vi "Generate Update Waveform.vi"(0 "updated signal in":refnum<class "SV Signal.lvclass">, 5 "previous signal":refnum<class "SV Signal.lvclass">, 7 "template waveform":waveform(dbl), 9 "samples":i32=1000, 11 "error in (no error)":errorcluster) -> (4 "updated signal out":refnum<class "SV Signal.lvclass">, 6 "previous signal out":refnum<class "SV Signal.lvclass">, 8 "output waveform":waveform(dbl), 10 "samples generated":i32=1000, 15 "error out":errorcluster)   [LabVIEW 2017, in "SV Signal.lvclass"]
uses:
  <vilib>/addons/_NISVFA/_Generation/Signal Generation/SV Signal/SV Signal.lvclass
  <vilib>/addons/_NISVFA/_Generation/Signal Generation/SV Signal/SV Signal.lvclass/SV Signal.ctl
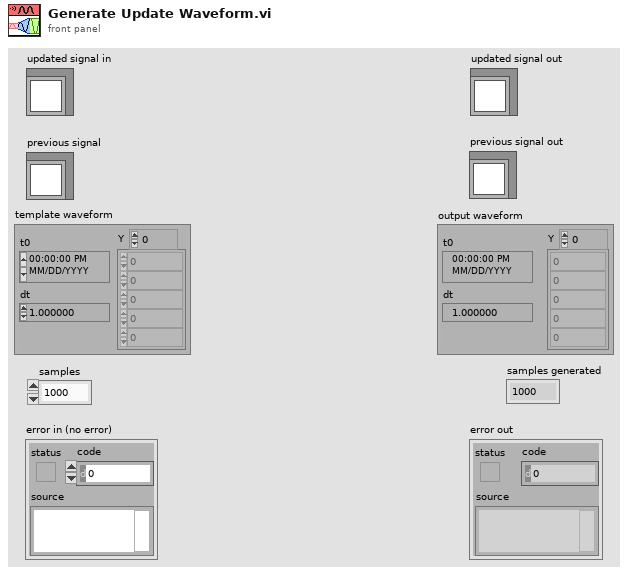
[diagram p1: front panel]
types:
  T1 = typedef "SV Signal.lvclass/sv_Generation State.ctl" = enum16{"Idle", "Ramp Up", "Pre-Measurement Settling", "Measurement", "Post-Measurement Settling", "Discrete Sweep Transition", "Ramp Down", "Update"}
  T2 = typedef "SV Signal.lvclass/sv_System Timing Model.ctl" = i64
  T3 = cluster{"system timing model":T2, "state":cluster{"RESET":bool, "generator timestamp":timestamp, "elapsed seconds":dbl, "elapsed samples":u64, "generation state":T1, "time offset at state":dbl, "samples generated at state":u64, "signal state":variant}, "duration of state":dbl, "samples remaining at state":i32}
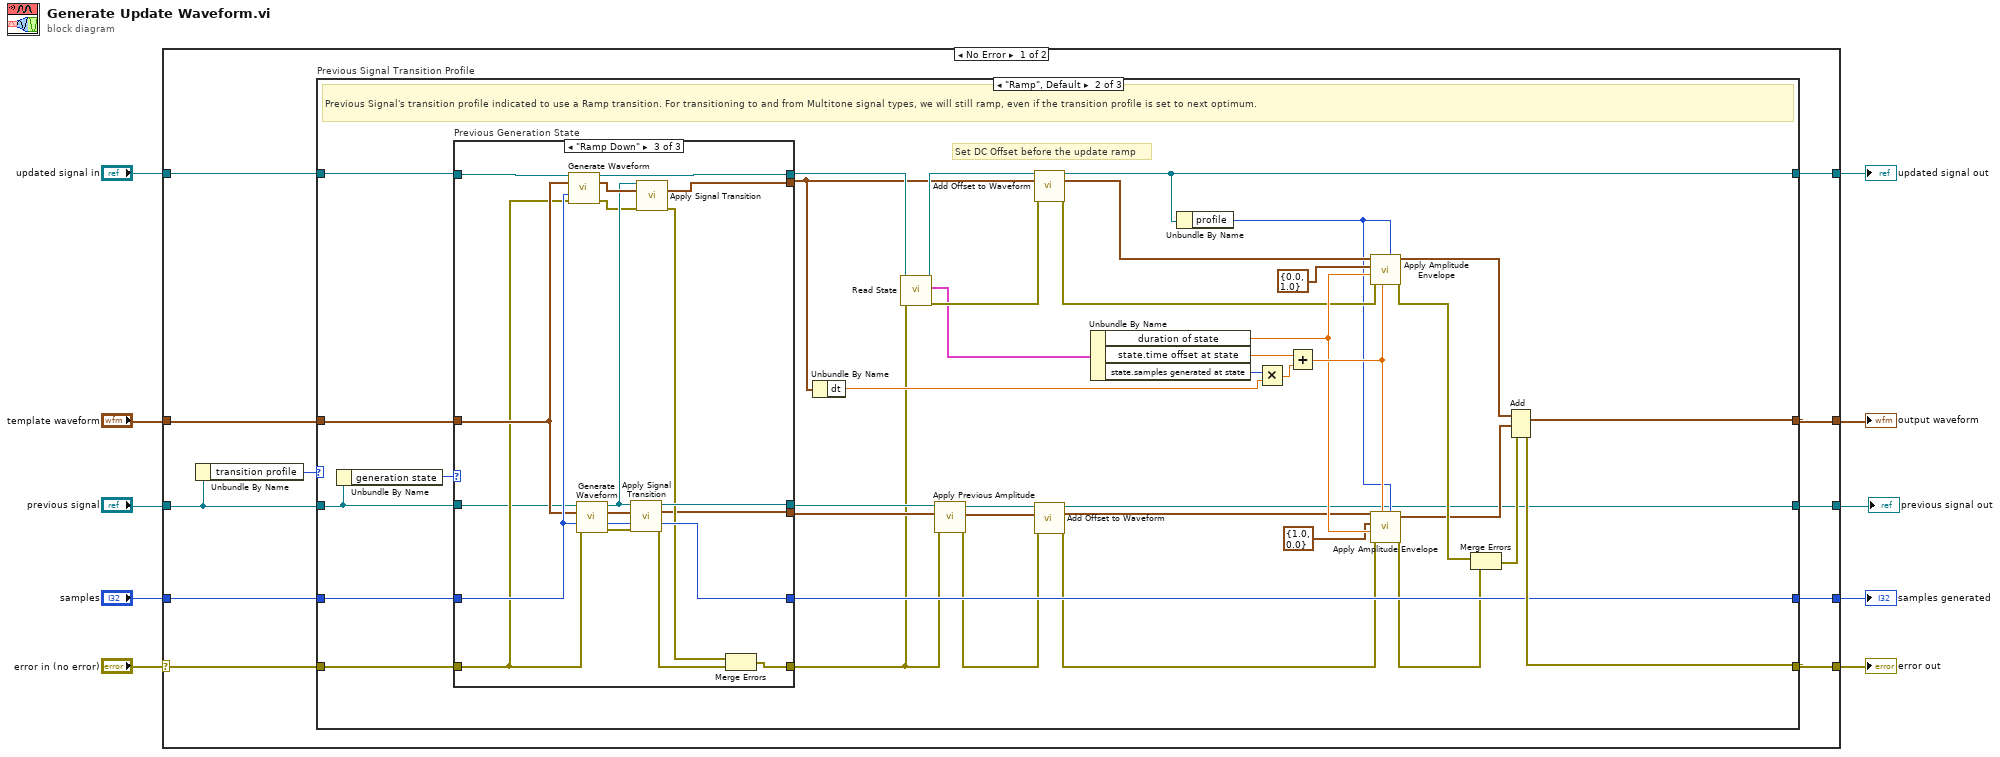
[diagram p0: block diagram]
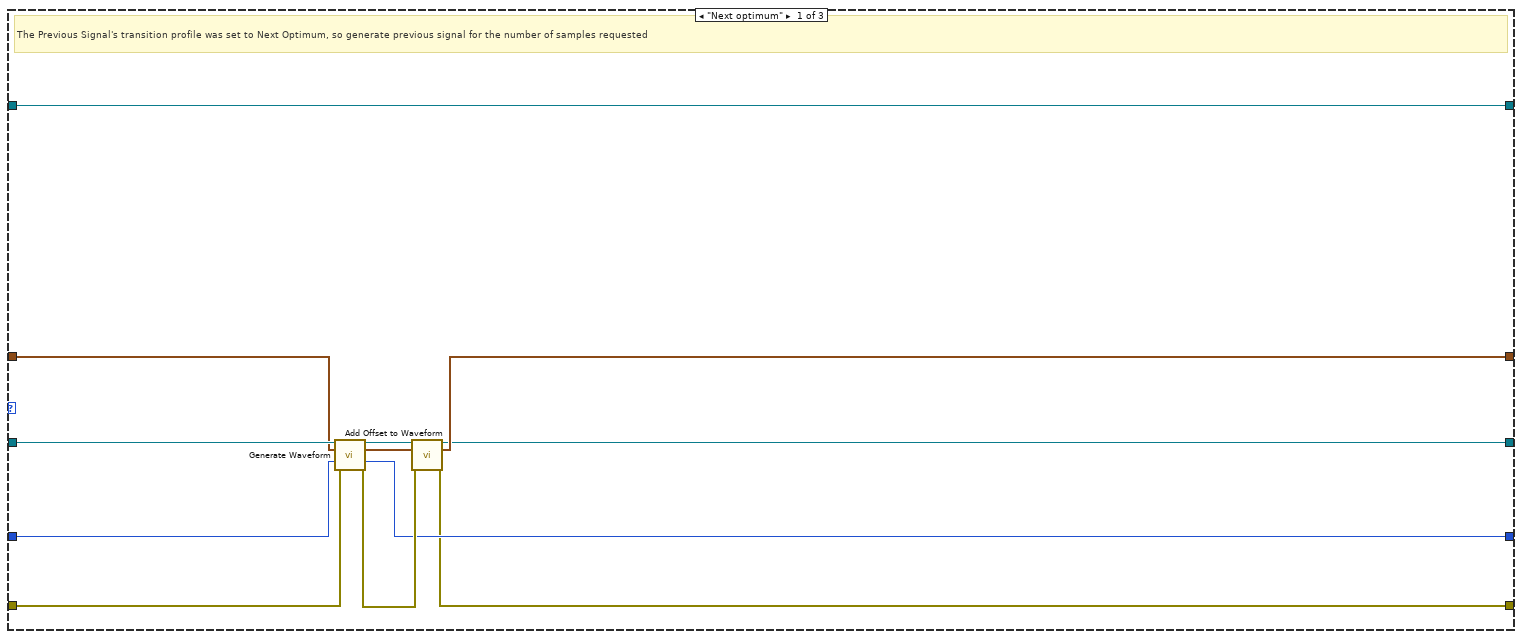
[diagram p2: hidden frame]
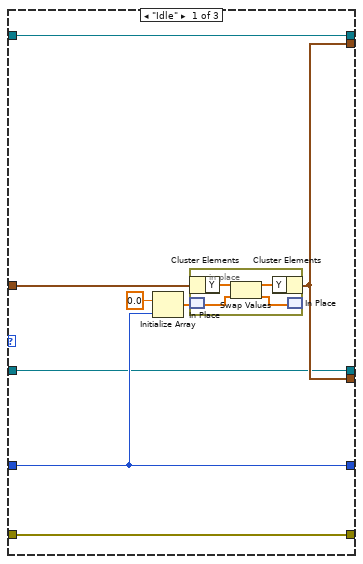
[diagram p3: hidden frame]
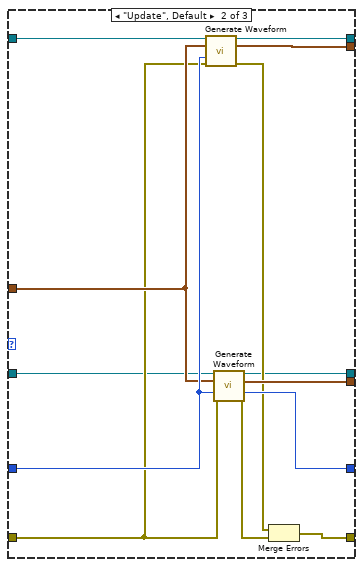
[diagram p4: hidden frame]
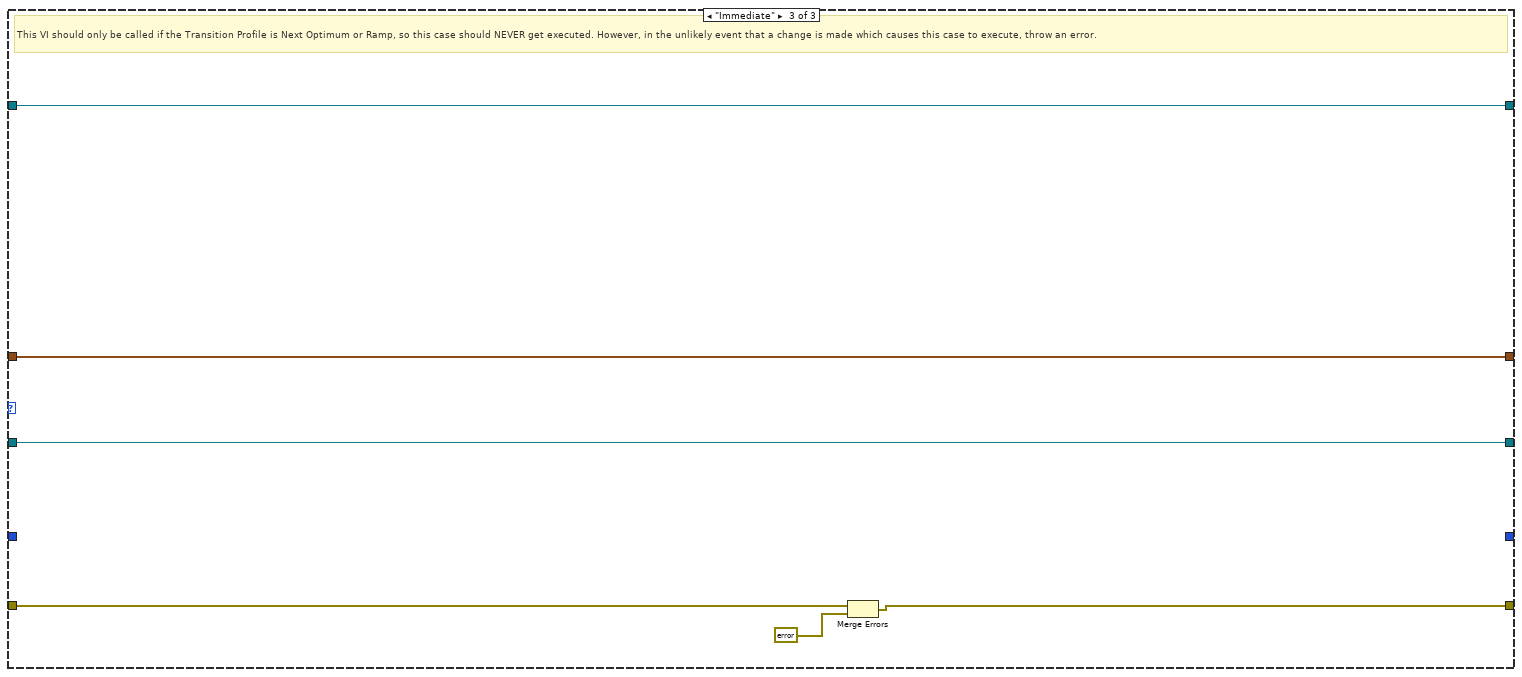
[diagram p5: hidden frame]
diagram:
  n1 = case shown="No Error" "error in (no error)" {
    selector: "error in (no error)" -> [w19 w126]
    tunnel: [w20 w126] -> w9
    tunnel: [w13 w125] -> w7
    tunnel: "updated signal in" -> [w21 w125]
    tunnel: [w18 _] -> w6
    tunnel: "samples" -> [w17 _]
    tunnel: "template waveform" -> [w16 w124]
    tunnel: "previous signal" -> [w15 w123]
    tunnel: [w14 w124] -> w2
    tunnel: [w11 w123] -> w1
    frame No Error {
      n2 = Unbundle By Name(w15) -> ("transition profile"=w12:enum16{"Immediate", "Next optimum", "Ramp"})
      n3 = case "Previous Signal Transition Profile" shown="\"Ramp\", Default" w12 {
        tunnel: w17 -> [w32 w73 _]
        tunnel: [w26 w72 w121] -> w14
        tunnel: [w22 w71 w119] -> w20
        tunnel: [w23 w35 w122] -> w13
        tunnel: w21 -> [w23 w69 w122]
        tunnel: w19 -> [w30 w68 w120]
        tunnel: [w25 w66 _] -> w18
        tunnel: w16 -> [w31 w65 w121]
        tunnel: w15 -> [w33 w64 w117]
        tunnel: [w24 w34 w117] -> w11
        frame "Next optimum" {
          # "The Previous Signal's transition profile was set to Next Optimum, so generate previous signal for the number of samples requested"
          n4 = call-dynamic "Generate Waveform.vi"("signal configuration and state in"=w33, "template waveform"=w31, "samples"=w32, "error in (no error)"=w30) -> ("signal configuration and state out"=w29:refnum<class "SV Signal.lvclass">, "output waveform"=w28:waveform(dbl), "samples"=w25:i32, "error out"=w27:errorcluster)  [unwired: 8 in]
          n5 = call <vilib>:"Add Offset to Waveform.vi"("signal configuration"=w29, "input waveform"=w28, "error in (no error)"=w27) -> ("signal configuration"=w24:refnum<class "SV Signal.lvclass">, "offset waveform"=w26:waveform(dbl), "error out"=w22:errorcluster)  [unwired: 9 in, 1 out]
        }
        frame "Ramp", Default {
          # "Set DC Offset before the update ramp"
          # "Previous Signal's transition profile indicated to use a Ramp transition. For transitioning to and from Multitone signal types, we will still ramp, even if the transition profile is set to next optimum."
          n6 = Unbundle By Name(w64) -> ("generation state"=w70:T1)
          n7 = case "Previous Generation State" shown="\"Ramp Down\"" w70 {
            tunnel: w69 -> [w75 w98 w116]
            tunnel: w73 -> [w77 w97 w115]
            tunnel: w65 -> [w81 w96 w114]
            tunnel: w68 -> [w76 w91 w111]
            tunnel: [w77 w95 w113] -> w66
            tunnel: [w78 w94 w104] -> w37
            tunnel: [w75 w93 w112] -> w67
            tunnel: [w76 w88 w110] -> w39
            tunnel: [w74 w86 w106] -> w43
            tunnel: [w78 w92 w99] -> w42
            tunnel: w64 -> [w74 w87 w109]
            frame "Idle" {
              n8 = Initialize Array(0.0 ("element"), w77) -> (w79:dbl[])
              n9 = in-place {
                n10 = in-place-cluster #1(w81) -> ("Y"=w85:dbl[])
                n11 = in-place-match #2(w79) -> (w83:dbl[])
                n12 = Swap Values(12:w85, 14:w83) -> (1:w84:dbl[], 3:w82:dbl[])  [unwired: 1 in]
                n13 = in-place-cluster #1("Y"=w84) -> (w78:waveform(dbl))
                n14 = in-place-match #2(w82) -> ()  [unwired: 1 out]
              }
            }
            frame "Update", Default {
              n15 = call-dynamic "Generate Waveform.vi"("signal configuration and state in"=w98, "template waveform"=w96, "samples"=w97, "error in (no error)"=w91) -> ("signal configuration and state out"=w93:refnum<class "SV Signal.lvclass">, "output waveform"=w94:waveform(dbl), "error out"=w89:errorcluster)  [unwired: 8 in, 1 out]
              n16 = call-dynamic "Generate Waveform.vi"("signal configuration and state in"=w87, "template waveform"=w96, "samples"=w97, "error in (no error)"=w91) -> ("signal configuration and state out"=w86:refnum<class "SV Signal.lvclass">, "output waveform"=w92:waveform(dbl), "samples"=w95:i32, "error out"=w90:errorcluster)  [unwired: 8 in]
              n17 = Merge Errors(w89, w90) -> (w88:errorcluster)
            }
            frame "Ramp Down" {
              n18 = call-dynamic "Generate Waveform.vi"("signal configuration and state in"=w116, "template waveform"=w114, "samples"=w115, "error in (no error)"=w111) -> ("signal configuration and state out"=w112:refnum<class "SV Signal.lvclass">, "output waveform"=w108:waveform(dbl), "error out"=w103:errorcluster)  [unwired: 8 in, 1 out]
              n19 = call-dynamic "Generate Waveform.vi"("signal configuration and state in"=w109, "template waveform"=w114, "samples"=w115, "error in (no error)"=w111) -> ("signal configuration and state out"=w107:refnum<class "SV Signal.lvclass">, "output waveform"=w105:waveform(dbl), "samples"=w113:i32, "error out"=w102:errorcluster)  [unwired: 8 in]
              n20 = call <vilib>:"Apply Signal Transition.vi"("signal configuration and state in"=w107, "waveform"=w105, "error in (no error)"=w102) -> ("signal configuration and state out"=w106:refnum<class "SV Signal.lvclass">, "profiled waveform"=w99:waveform(dbl), "error out"=w101:errorcluster)  [unwired: 10 in]
              n21 = call <vilib>:"Apply Signal Transition.vi"("signal configuration and state in"=w107, "waveform"=w108, "error in (no error)"=w103) -> ("profiled waveform"=w104:waveform(dbl), "error out"=w100:errorcluster)  [unwired: 10 in, 1 out]
              n22 = Merge Errors(w100, w101) -> (w110:errorcluster)
            }
          }
          n23 = Unbundle By Name(w37) -> ("dt"=w62:dbl)
          n24 = call <vilib>:"Read State.vi"("error in (no error)"=w39, "signal configuration"=w67) -> ("error out"=w47:errorcluster, "generator state"=w46:T3, "signal configuration"=w48:refnum<class "SV Signal.lvclass">)  [unwired: 7 in]
          n25 = call <vilib>:"Apply Previous Amplitude.vi"("error in (no error)"=w39, "waveform in"=w42, "SV Signal in"=w43) -> ("error out"=w38:errorcluster, "waveform out"=w40:waveform(dbl), "SV Signal out"=w41:refnum<class "SV Signal.lvclass">)  [unwired: 6 in]
          n26 = call <vilib>:"Add Offset to Waveform.vi"("signal configuration"=w48, "input waveform"=w37, "error in (no error)"=w47) -> ("signal configuration"=w35:refnum<class "SV Signal.lvclass">, "offset waveform"=w53:waveform(dbl), "error out"=w54:errorcluster)  [unwired: 9 in, 1 out]
          n27 = call <vilib>:"Add Offset to Waveform.vi"("signal configuration"=w41, "input waveform"=w40, "error in (no error)"=w38) -> ("signal configuration"=w34:refnum<class "SV Signal.lvclass">, "offset waveform"=w44:waveform(dbl), "error out"=w45:errorcluster)  [unwired: 9 in, 1 out]
          n28 = Unbundle By Name(w46) -> ("duration of state"=w57:dbl, "state.time offset at state"=w59:dbl, "state.samples generated at state"=w61:u64)
          n29 = Unbundle By Name(w35) -> ("profile"=w36:enum16{"Linear", "Half cosine"})
          n30 = Multiply(x=w61, y=w62) -> (x*y=w60:dbl)
          n31 = Add(x=w59, y=w60) -> (x+y=w58:dbl)
          n32 = call <vilib>:"Apply Amplitude Envelope.vi"("profile"=w36, "time elapsed at transition"=w58, "error in (no error)"=w54, "duration"=w57, "amplitude modulation"=cluster{"start":dbl, "stop":dbl} {"start"=0.0, "stop"=1.0}, "waveform in"=w53) -> ("error out"=w51:errorcluster, "waveform out"=w52:waveform(dbl))  [unwired: 3 in, 1 out]
          n33 = call <vilib>:"Apply Amplitude Envelope.vi"("profile"=w36, "time elapsed at transition"=w58, "error in (no error)"=w45, "duration"=w57, "amplitude modulation"=cluster{"start":dbl, "stop":dbl} {"start"=1.0, "stop"=0.0}, "waveform in"=w44) -> ("error out"=w50:errorcluster, "waveform out"=w49:waveform(dbl))  [unwired: 3 in, 1 out]
          n34 = Merge Errors(w51, w50) -> (w55:errorcluster)
          n35 = Add(1:w49, 2:w52, 4:w55) -> (0:w72:waveform(dbl), 3:w71:errorcluster)
        }
        frame "Immediate" {
          # "This VI should only be called if the Transition Profile is Next Optimum or Ramp, so this case should NEVER get executed. However, in the unlikely event that a change is made which causes this case to execute, throw an error."
          n36 = Merge Errors(w120, errorcluster {"status"=TRUE, "code"=-1984, "source"="It should not be possible for this error to occur. Please contact NI if you receive this error and ask to speak to the Sound & Vibration team "} ("error in")) -> (w119:errorcluster)
        }
      }
    }
    frame Error {
    }
  }
  "error out" <- w9
  "updated signal out" <- w7
  "output waveform" <- w2
  "samples generated" <- w6
  "previous signal out" <- w1
